vi "CopyVI.vi"(8 "error in (no error)":errorcluster, 9 "application reference (local)":refnum<vi>, 10 "Empty File":path=path "D:/Git/CSPP_MessageMaker/_CSPP_MessageMaker/TestVIs/TestTarget.vi", 11 "File to Copy":path) -> (0 "error out":errorcluster)   [LabVIEW 2014, in "CS++Actor.lvlib" / "CS++Actor.lvclass"]
uses:
  CS++Actor.lvclass
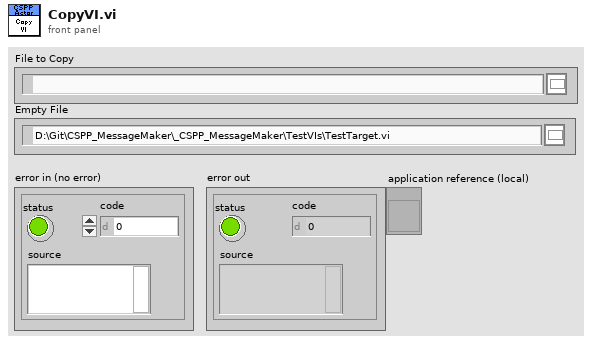
[diagram p1: front panel]
types:
  T1 = enum16{"Invalid Wire Rule", "Required", "Recommended", "Optional", "Dynamic Dispatch"}
  T2 = enum16{"Invalid Wire Rule", "Required", "Recommended", "Optional", "Dynamic Dispatch"}[]
  T3 = typedef "LVPositionTypeDef.ctl" = cluster{"Left":i32, "Top":i32}
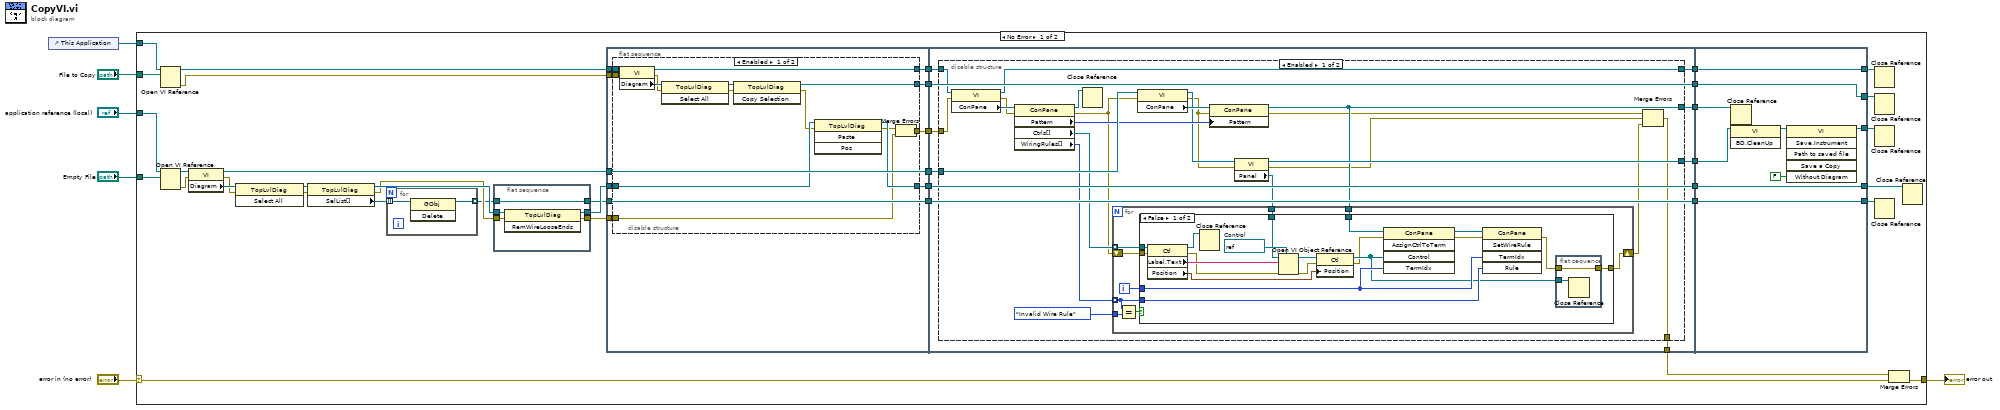
[diagram p0: block diagram]
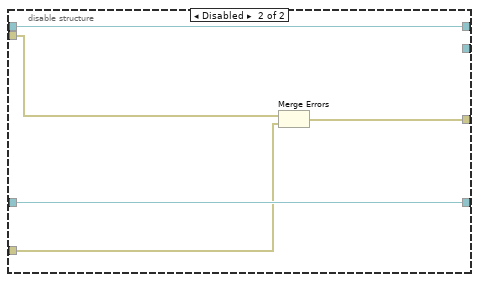
[diagram p2: hidden frame]
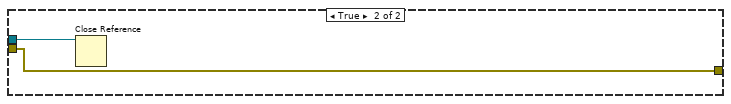
[diagram p3: hidden frame]
diagram:
  n1 = control-ref of="This Application"() -> (w1:refnum<vi>)
  n2 = case shown="No Error" "error in (no error)" {
    selector: "error in (no error)" -> [w18 w158]
    tunnel: [w17 w158] -> w5
    tunnel: "File to Copy" -> [w10 _]
    tunnel: "Empty File" -> [w12 _]
    tunnel: "application reference (local)" -> [w8 _]
    tunnel: w1 -> [w7 _]
    frame No Error {
      n3 = Open VI Reference(application reference (local)=w7, vi path=w10) -> (vi reference=w9:refnum<vi>, error out=w11:errorcluster)  [unwired: 4 in]
      n4 = Open VI Reference(application reference (local)=w8, vi path=w12) -> (vi reference=w35:refnum<vi>, error out=w30:errorcluster)  [unwired: 4 in]
      n5 = property class="VI"(reference=w35, error in=w30) -> (reference out=w29:refnum<vi>, error out=w33:errorcluster, "Diagram"=w34:refnum<vi>)
      n6 = invoke class="TopLvlDiag" method="Select All"(reference=w34, error in=w33) -> (reference out=w32:refnum<vi>, error out=w31:errorcluster)  [unwired: 1 in, 1 out]
      n7 = property class="TopLvlDiag"(reference=w32, error in=w31) -> (reference out=w23:refnum<vi>, error out=w15:errorcluster, "SelList[]"=w21:refnum<vi>[])
      n8 = for {
        tunnel: w21 -> [w157] mode=indexing
        tunnel: [w156] -> w13 mode=indexing
        n9 = invoke class="GObj" method="Delete"(reference=w157) -> (reference out=w156:refnum<vi>)  [unwired: 2 in, 2 out]
      }
      n10 = flat-sequence {
        tunnel: w23 -> [w51]
        tunnel: [w50] -> w22
        tunnel: [w49] -> w20
        tunnel: w15 -> [w48]
        tunnel: [w47] -> w14
        tunnel: w13 -> [w47]
        frame #0 {
          n11 = invoke class="TopLvlDiag" method="RemWireLooseEnds"(reference=w51, error in=w48) -> (reference out=w50:refnum<vi>, error out=w49:errorcluster)  [unwired: 1 in, 1 out]
        }
      }
      n12 = flat-sequence {
        tunnel: w9 -> [w61]
        tunnel: w11 -> [w60]
        tunnel: w22 -> [w57]
        tunnel: w14 -> [w59]
        tunnel: w29 -> [w58]
        tunnel: [w56] -> w46
        tunnel: [w59] -> w45
        tunnel: [w58] -> w44
        tunnel: [w55] -> w43
        tunnel: [w53] -> w42
        tunnel: w20 -> [w54]
        tunnel: [w52] -> w19
        tunnel: w46 -> [w87]
        tunnel: [w87] -> w41
        tunnel: w45 -> [w90]
        tunnel: [w90] -> w40
        tunnel: w44 -> [w86]
        tunnel: [w85] -> w39
        tunnel: w43 -> [w88]
        tunnel: [w81] -> w38
        tunnel: w42 -> [w89]
        tunnel: [w89] -> w37
        tunnel: [w84] -> w36
        tunnel: w19 -> [w83]
        tunnel: [w82] -> w16
        tunnel: [w154] -> w27
        tunnel: [w155] -> w28
        tunnel: w41 -> [w155]
        tunnel: w40 -> [w154]
        tunnel: w39 -> [w152]
        tunnel: [w151] -> w26
        tunnel: [w150] -> w25
        tunnel: w38 -> [w150]
        tunnel: [w149] -> w24
        tunnel: w37 -> [w149]
        tunnel: w36 -> [w148]
        frame #0 {
          n13 = disable-structure shown="Enabled" {
            disable-tunnel: w61 -> [w75 w80]
            disable-tunnel: w60 -> [w74 w79]
            disable-tunnel: w57 -> [w69 w78]
            disable-tunnel: [w68 w78] -> w56
            disable-tunnel: [w66 w80] -> w55
            disable-tunnel: w54 -> [w65 w76]
            disable-tunnel: [w63 _] -> w53
            disable-tunnel: [w64 w77] -> w52
            frame Enabled {
              n14 = property class="VI"(reference=w75, error in=w74) -> (reference out=w66:refnum<vi>, error out=w72:errorcluster, "Diagram"=w73:refnum<vi>)
              n15 = invoke class="TopLvlDiag" method="Select All"(reference=w73, error in=w72) -> (reference out=w71:refnum<vi>, error out=w70:errorcluster)  [unwired: 1 in, 1 out]
              n16 = invoke class="TopLvlDiag" method="Copy Selection"(reference=w71, error in=w70) -> (reference out=w63:refnum<vi>, error out=w67:errorcluster)  [unwired: 1 in, 1 out]
              n17 = invoke class="TopLvlDiag" method="Paste"(reference=w69, error in=w67) -> (reference out=w68:refnum<vi>, error out=w62:errorcluster)  [unwired: 2 in, 2 out]
              n18 = Merge Errors(w62, w65) -> (w64:errorcluster)
            }
            frame Disabled {
              n19 = Merge Errors(w79, w76) -> (w77:errorcluster)
            }
          }
        }
        frame #1 {
          n20 = disable-structure shown="Enabled" {
            disable-tunnel: w88 -> [w111 w146]
            disable-tunnel: w86 -> [w109 w145]
            disable-tunnel: [w103 w145] -> w85
            disable-tunnel: [w101 _] -> w84
            disable-tunnel: w83 -> [w100 _]
            disable-tunnel: [w93 _] -> w82
            disable-tunnel: [w91 w146] -> w81
            frame Enabled {
              n21 = property class="VI"(reference=w111, error in=w100) -> (reference out=w91:refnum<vi>, error out=w99:errorcluster, "ConPane"=w112:refnum<vi>)
              n22 = property class="ConPane"(reference=w112, error in=w99) -> (reference out=w108:refnum<vi>, error out=w97:errorcluster, "Pattern"=w107:u32, "Ctrls[]"=w106:refnum<vi>[], "WiringRules[]"=w105:T2)
              n23 = Close Reference(reference=w108) -> ()  [unwired: 1 in, 1 out]
              n24 = property class="VI"(reference=w109, error in=w97) -> (reference out=w104:refnum<vi>, error out=w98:errorcluster, "ConPane"=w110:refnum<vi>)
              n25 = property class="ConPane"(reference=w110, error in=w98, "Pattern"=w107) -> (reference out=w101:refnum<vi>, error out=w94:errorcluster)
              n26 = property class="VI"(reference=w104, error in=w98) -> (reference out=w103:refnum<vi>, error out=w95:errorcluster, "Panel"=w102:refnum<vi>)
              n27 = for {
                tunnel: w106 -> [w121] mode=indexing
                tunnel: w105 -> [w115] mode=indexing
                tunnel: w102 -> [w120]
                tunnel: w101 -> [w119]
                shift-right: [w117] -> w96
                shift-left: w97 -> [w118]
                tunnel: T1."Invalid Wire Rule" ("Wire Rule") -> [w113]
                i -> [w116]
                n28 = Equal?(x=w115, y=w113) -> (x = y?=w114:bool)
                n29 = case shown="False" w114 {
                  tunnel: w121 -> [w140 w144]
                  tunnel: w120 -> [w137 _]
                  tunnel: w119 -> [w132 _]
                  tunnel: w116 -> [w131 _]
                  tunnel: w115 -> [w130 _]
                  tunnel: w118 -> [w127 w143]
                  tunnel: [w122 w143] -> w117
                  frame False {
                    w138 = refnum<vi> refnum  # Control
                    n30 = property class="Ctl"(reference=w140, error in=w127) -> (reference out=w139:refnum<vi>, error out=w126:errorcluster, "Label.Text"=w136:string, "Position"=w134:T3)
                    n31 = Close Reference(reference=w139) -> ()  [unwired: 1 in, 1 out]
                    n32 = Open VI Object Reference(7:w138, 8:w126, 10:w136, 11:w137) -> (0:w125:errorcluster, 3:w135:refnum<vi>)
                    n33 = property class="Ctl"(reference=w135, error in=w125, "Position"=w134) -> (reference out=w129:refnum<vi>, error out=w124:errorcluster)
                    n34 = invoke class="ConPane" method="AssignCtrlToTerm"(reference=w132, error in=w124, "Control"=w129, "TermIdx"=w131) -> (reference out=w133:refnum<vi>, error out=w123:errorcluster)  [unwired: 1 in, 3 out]
                    n35 = invoke class="ConPane" method="SetWireRule"(reference=w133, error in=w123, "TermIdx"=w131, "Rule"=w130) -> (error out=w128:errorcluster)  [unwired: 1 in, 4 out]
                    n36 = flat-sequence {
                      tunnel: w129 -> [w142]
                      tunnel: w128 -> [w141]
                      tunnel: [w141] -> w122
                      frame #0 {
                        n37 = Close Reference(reference=w142) -> ()  [unwired: 1 in, 1 out]
                      }
                    }
                  }
                  frame True {
                    n38 = Close Reference(reference=w144) -> ()  [unwired: 1 in, 1 out]
                  }
                }
              }
              n39 = Merge Errors(w94, w95, w96) -> (w93:errorcluster)
            }
            frame Disabled {
            }
          }
        }
        frame #2 {
          n40 = Close Reference(reference=w148) -> ()  [unwired: 1 in, 1 out]
          n41 = invoke class="VI" method="BD.CleanUp"(reference=w152) -> (reference out=w153:refnum<vi>)  [unwired: 2 in, 2 out]
          n42 = invoke class="VI" method="Save.Instrument"(reference=w153, "Without Diagram"=FALSE) -> (reference out=w151:refnum<vi>)  [unwired: 4 in, 5 out]
        }
      }
      n43 = Close Reference(reference=w25) -> ()  [unwired: 1 in, 1 out]
      n44 = Close Reference(reference=w24) -> ()  [unwired: 1 in, 1 out]
      n45 = Close Reference(reference=w26) -> ()  [unwired: 1 in, 1 out]
      n46 = Close Reference(reference=w27) -> ()  [unwired: 1 in, 1 out]
      n47 = Merge Errors(w16, w18) -> (w17:errorcluster)
      n48 = Close Reference(reference=w28) -> ()  [unwired: 1 in, 1 out]
    }
    frame Error {
    }
  }
  "error out" <- w5
